vi "Configure Branch Limit Dynamic.vi"(5 "Limit Type (0: Above)":i32(ring) items=["Above", "Below", "Inside", "Outside"], 6 "Measure Block (0)":u32, 7 "Limit Number (1: Limit Number 1)":i32(ring)=1 items=["Limit Number 1"=1, "Limit Number 2"=2], 8 "error in (no error)":errorcluster, 9 "Branch To Block (0)":u32, 10 "Block Number (1)":u32=1, 11 "VISA resource name":refnum<visa-resource-name>) -> (0 "error out":errorcluster, 3 "VISA resource name out":refnum<visa-resource-name>)   [LabVIEW 2023, in "Keithley DMM6500 DAQ6500 Series.lvlib"]
doc: "Defines a trigger model block that goes to a specified block in the trigger model if a measurement meets user-defined criteria."
uses:
  <instrlib>/Keithley DMM6500 DAQ6500 Series/Keithley DMM6500 DAQ6500 Series.lvlib
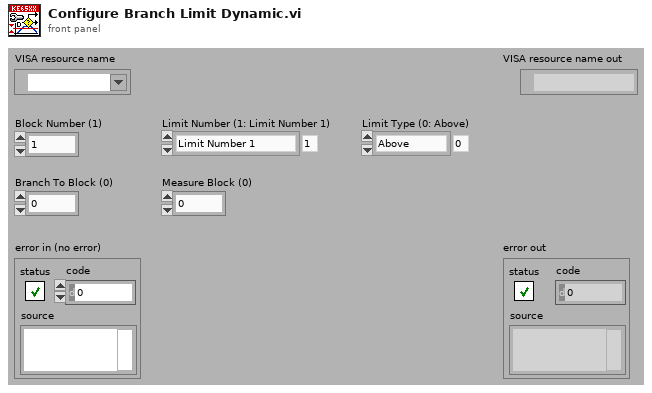
[diagram p1: front panel]
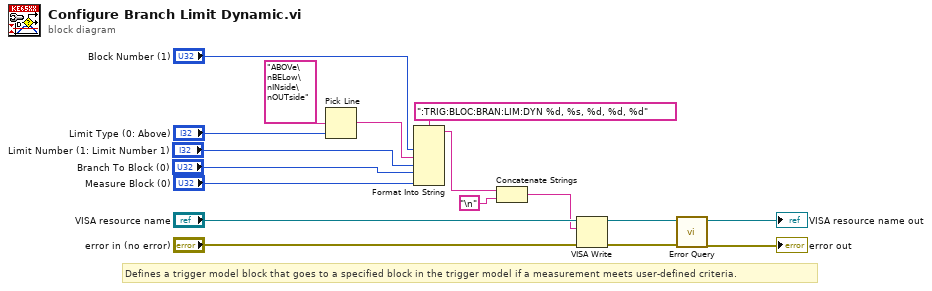
[diagram p0: block diagram]
diagram:
  # "Defines a trigger model block that goes to a specified block in the trigger model if a measurement meets user-defined criteria."
  n1 = Pick Line(multi-line string="ABOVe\nBELow\nINside\nOUTside", line index="Limit Type (0: Above)") -> (output string=w3:string)  [unwired: 1 in]
  n2 = Format Into String(format string=":TRIG:BLOC:BRAN:LIM:DYN %d, %s, %d, %d, %d", "Block Number (1)", w3, "Limit Number (1: Limit Number 1)", "Branch To Block (0)", "Measure Block (0)") -> (resulting string=w4:string)  [unwired: 2 in, 1 out]
  n3 = Concatenate Strings(w4, "\n") -> (w6:string)
  n4 = VISA Write(VISA resource name="VISA resource name", write buffer=w6, error in (no error)="error in (no error)") -> (VISA resource name out=w12:refnum<visa-resource-name>, error out=w11:errorcluster)  [unwired: 1 out]
  n5 = call <instrlib>:"Error Query.vi"("error in (no error)"=w11, "VISA resource name"=w12) -> ("error out"=→"error out":errorcluster, "VISA resource name out"=→"VISA resource name out":refnum<visa-resource-name>)  [unwired: 6 in, 2 out]
